vi "CPP-6compBalance.vi"() -> (5 "Plug in titles":string[](array[string]), 7 "Plug in values":string[](array[string]))   [LabVIEW 2022 SP3]
uses:
  <vilib>/Analysis/baseanly.llb/A x Vector.vi
  <vilib>/Analysis/8numeric.llb/1D Numeric Integration.vi
  Globals/Meas_global.vi
  <vilib>/Analysis/NI_AALBase.lvlib
  <vilib>/Analysis/NI_AALPro.lvlib
panel:
  out "welchStyle":cluster{"f0":dbl, "df":dbl, "PSD(f)":dbl[]}[](graph)
  out "x/y":dbl[](array[numeric])
  out "Integrals":dbl[](array[numeric])
  out "ensembleByBlock":dbl[][](graph)
  out "SDs":dbl[](array[numeric])
  out "means":dbl[](array[numeric])
  out "calibrated":dbl[][](array[numeric])
  out "Eng Values":dbl[][](array[numeric])
  out "calibArray":dbl[][](array[numeric])
  in  "ATI Cal File":path
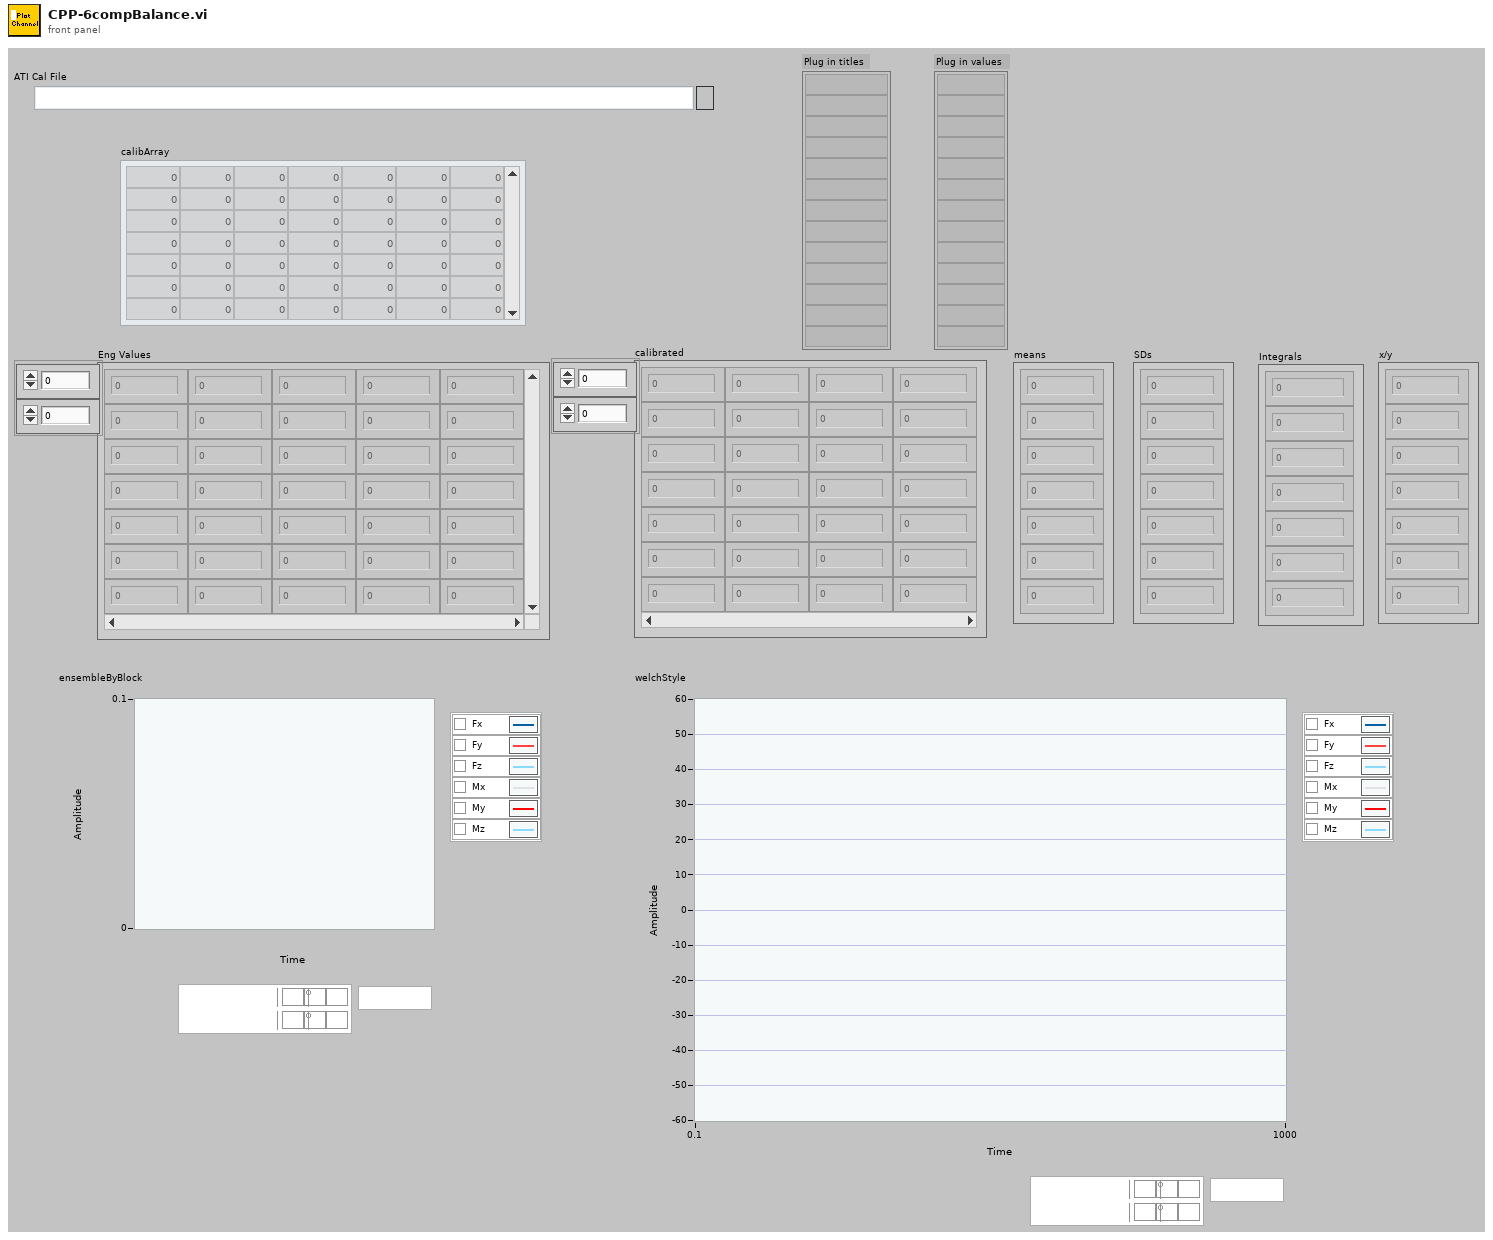
[diagram p1: front panel]
types:
  T1 = typedef "Analysis_info_cluster.ctl" = cluster{"Colour":u32, "Inst type":T2, "Inst name":string, "Symbol":string, "Code name":string, "Extra Info":string, "Inst Array":T3, "Extra Titles":string[], "Extra Values":string[], "U":dbl, "u^2":dbl, "u^3":dbl, "u^4":dbl, "Skew_u":dbl, "Kurt_u":dbl, "Sd Error in Mean":dbl, "% u'/U":dbl, "X":dbl, "Y":dbl, "Z":dbl, "Timescale integral Estimate":dbl, "Sd Error in Variance":dbl, "Calib File":path, "Calib Constants":dbl[], "Output Position":bool, "Stats":enum16{"None", "Basic", "Full"}, "Av Sampling Rate":dbl, "Av No of Samples":dbl, "Total Meas Time (s)":dbl, "ADAM Ch Name":string, "Max value":dbl, "Min value":dbl, "Req Sample Rate Hz":dbl, "Sync Delay Time (s)":dbl, "Ch No":i16, "Device":string, "Use Latest Calib":bool, "Port":string, "Metadata Ch Names":string[], "Metadata Ch Values":string[], "Label":string}
  T2 = typedef "Inst_type.ctl" = enum16{"Raw voltage", "Raw with zero offsetting", "Propeller anemometer", "Pressure Transducer", "Pitot-static tube", "Hot wire", "Cross wire 1", "Cross wire 2", "Generic Linear", "Generic Polynomial", "Generic BackPoly", "Fast FID", "Thermocouple", "Cold wire", "Pulsed Wire", "LDA Vel", "LDA Tran time", "LDA Arr time", "Microphone"}
  T3 = typedef "Instrument_Array.ctl" = enum16{"PWA", "LDA", "Analogue"}
  T4 = typedef "Time_Trace_Cluster.ctl" = cluster{"Weighting":dbl[], "Voltage":dbl[], "Eng Values":dbl[]}
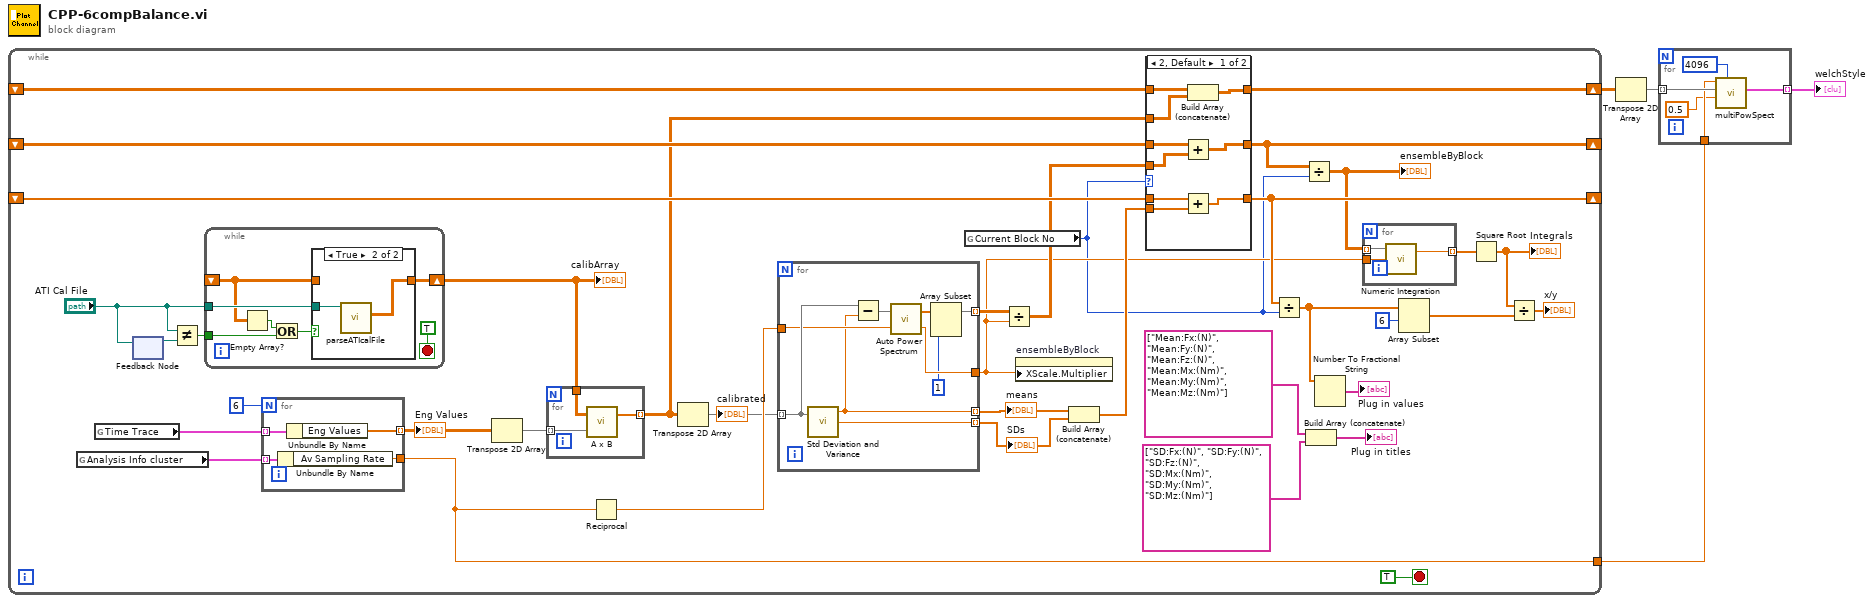
[diagram p0: block diagram]
diagram:
  n1 = while {
    shift-right: [w20] -> _
    shift-left: _ -> [w34]
    shift-right: [w12] -> _
    shift-left: _ -> [w27]
    shift-right: [w9] -> w4
    shift-left: _ -> [w8]
    tunnel: [w7] -> w3
    stop <- TRUE stop-if-true
    n2 = global read "Meas_global.vi" "Analysis Info cluster"() -> (w41:T1[])
    n3 = global read "Meas_global.vi" "Time Trace"() -> (w42:T4[])
    n4 = feedback-in #1("ATI Cal File") -> ()
    n5 = feedback #1() -> (w30:path)  [unwired: 1 in]
    n6 = Not Equal?(x="ATI Cal File", y=w30) -> (x != y?=w28:bool)
    n7 = while {
      shift-right: [w64] -> w37
      shift-left: _ -> [w60]
      tunnel: "ATI Cal File" -> [w62]
      tunnel: w28 -> [w58]
      stop <- TRUE stop-if-true
      n8 = Empty Array?(array=w60) -> (empty?=w61:bool)
      n9 = Or(x=w61, y=w58) -> (x .or. y?=w59:bool)
      n10 = case shown="True" w59 {
        tunnel: w62 -> [_ w66]
        tunnel: [w65 w67] -> w64
        tunnel: w60 -> [w65 _]
        frame False {
        }
        frame True {
          n11 = call "parseATIcalFile.vi"("Calibration File"=w66) -> ("Calibration array"=w67:dbl[][])  [unwired: 9 in, 1 out]
        }
      }
    }
    "calibArray" <- w37
    n12 = for {
      N: 6 -> [_]
      tunnel: w42 -> [w83] mode=indexing
      tunnel: [w82] -> w40 mode=indexing
      tunnel: w41 -> [w81] mode=indexing
      tunnel: [w80] -> w7
      n13 = Unbundle By Name(w81) -> ("Av Sampling Rate"=w80:dbl)
      n14 = Unbundle By Name(w83) -> ("Eng Values"=w82:dbl[])
    }
    "Eng Values" <- w40
    n15 = Transpose 2D Array(2D array=w40) -> (transposed array=w39:dbl[][])
    n16 = for {
      tunnel: w37 -> [w79]
      tunnel: w39 -> [w78] mode=indexing
      tunnel: [w77] -> w6 mode=indexing
      n17 = call-poly <vilib>:"A x B.vi"("Vector"=w78, "A"=w79) -> ("A x Vector"=w77:dbl[])  [unwired: 1 out]
    }
    n18 = Reciprocal(x=w7) -> (1/x=w24:dbl)
    n19 = Transpose 2D Array(2D array=w6) -> (transposed array=w10:dbl[][])
    "calibrated" <- w10
    n20 = for {
      tunnel: w10 -> [w75] mode=indexing
      tunnel: [w70] -> w36 mode=indexing
      tunnel: [w76] -> w22 mode=indexing
      tunnel: w24 -> [w74]
      tunnel: [w69] -> w23 mode=indexing
      tunnel: [w73] -> w13
      n21 = call <vilib>:"Std Deviation and Variance.vi"("X"=w75) -> ("mean"=w70:dbl, "standard deviation"=w76:dbl)  [unwired: 1 in, 1 out]
      n22 = Subtract(x=w75, y=w70) -> (x-y=w71:dbl[])
      n23 = call <vilib>:"Auto Power Spectrum.vi"("dt"=w74, "Signal (V)"=w71) -> ("df"=w73:dbl, "Power Spectrum (V^2 rms)"=w72:dbl[])
      n24 = Array Subset(array=w72, index=1) -> (w69:dbl[])  [unwired: 1 in]
    }
    "means" <- w36
    "SDs" <- w22
    n25 = global read "Meas_global.vi" "Current Block No"() -> (w11:i32)
    n26 = Divide(x=w23, y=w13) -> (x/y=w14:dbl[][])
    n27 = property on="ensembleByBlock" class="WFGraph (strict)"("XScale.Multiplier"=w13) -> ()  [unwired: 2 in, 2 out]
    n28 = Build Array (concatenate)(w36, w22) -> (w35:dbl[])
    n29 = case shown="2, Default" w11 {
      tunnel: [w54 w57] -> w20
      tunnel: w35 -> [w53 w57]
      tunnel: w34 -> [w52 _]
      tunnel: [w51 w56] -> w12
      tunnel: w14 -> [w50 w56]
      tunnel: w27 -> [w49 _]
      tunnel: [w46 w55] -> w9
      tunnel: w6 -> [w48 w55]
      tunnel: w8 -> [w47 _]
      frame 2, Default {
        n30 = Add(x=w49, y=w50) -> (x+y=w51:dbl[][])
        n31 = Add(x=w52, y=w53) -> (x+y=w54:dbl[])
        n32 = Build Array (concatenate)(w47, w48) -> (w46:dbl[][])
      }
      frame 1 {
      }
    }
    n33 = Divide(x=w20, y=w11) -> (x/y=w17:dbl[])
    n34 = Divide(x=w12, y=w11) -> (x/y=w5:dbl[][])
    "ensembleByBlock" <- w5
    n35 = Build Array (concatenate)(string[] ["Mean:Fx:(N)", "Mean:Fy:(N)", "Mean:Fz:(N)", "Mean:Mx:(Nm)", "Mean:My:(Nm)", "Mean:Mz:(Nm)"] ("Plug in titles"), string[] ["SD:Fx:(N)", "SD:Fy:(N)", "SD:Fz:(N)", "SD:Mx:(Nm)", "SD:My:(Nm)", "SD:Mz:(Nm)"] ("Plug in titles")) -> (→"Plug in titles":string[])
    n36 = Number To Fractional String(number=w17) -> (F-format string=→"Plug in values":string[])  [unwired: 3 in]
    n37 = for {
      tunnel: w5 -> [w45] mode=indexing
      tunnel: [w44] -> w15 mode=indexing
      tunnel: w13 -> [w43]
      n38 = call-poly <vilib>:"Numeric Integration.vi"("dt"=w43, "Input Array"=w45) -> ("result"=w44:dbl)  [unwired: 1 in, 1 out]
    }
    n39 = Array Subset(array=w17, index=6) -> (w19:dbl[])  [unwired: 1 in]
    n40 = Square Root(x=w15) -> (sqrt(x)=w16:dbl[])
    "Integrals" <- w16
    n41 = Divide(x=w16, y=w19) -> (x/y=→"x/y":dbl[])
  }
  n42 = Transpose 2D Array(2D array=w4) -> (transposed array=w2:dbl[][])
  n43 = for {
    tunnel: w2 -> [w88] mode=indexing
    tunnel: w3 -> [w87]
    tunnel: [w86] -> w1 mode=indexing
    n44 = call "multiPowSpect.vi"("subLength"=4096, "overlap(0- 0.9)"=0.5, "timeseries"=w88, "samplingFrequency"=w87) -> ("PSDdB"=w86:cluster{"f0":dbl, "df":dbl, "PSD(f)":dbl[]})  [unwired: 5 in, 2 out]
  }
  "welchStyle" <- w1
